vi "SetMode2.vi"() -> (0 "output cluster":T1 {"Och" format="%x"; "invrt" format="%x"; "Outdrv" format="%x"; "Outne_1" format="%x"; "Outne_0" format="%x"})   [LabVIEW 2022 SP3, in "PCA9685.lvlib" / "PCA.lvclass"]
uses:
  PCA.lvclass
  typedefs/Mode2.ctl
  PCA.lvclass/PCA.ctl
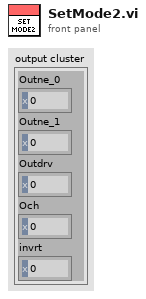
[diagram p1: front panel]
types:
  T1 = typedef "PCA9685.lvlib/PCA.lvclass/Mode2.ctl" = cluster{"Outne_0":u8, "Outne_1":u8, "Outdrv":u8, "invrt":u8, "Och":u8}
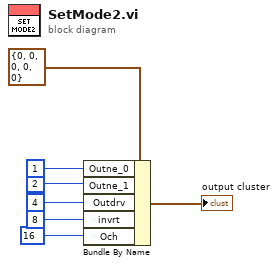
[diagram p0: block diagram]
diagram:
  n1 = Bundle By Name(cluster=T1 {"Outne_0"=0, "Outne_1"=0, "Outdrv"=0, "invrt"=0, "Och"=0} ("Mode2"), "Outne_0"=u8 1 ("Allcall"), "Outne_1"=u8 2 ("Allcall"), "Outdrv"=u8 4 ("Allcall"), "invrt"=u8 8 ("Allcall"), "Och"=u8 16 ("Allcall")) -> (→"output cluster":T1)
